vi "Stellglied.vi"(8 "error in (no error)":errorcluster caption="Fehler (Eingang, kein Fehler)", 10 "Stellgröße - Kraft (N)":dbl, 11 "RPDO2 object in":refnum<k20>) -> (0 "error out":errorcluster caption="Fehler (Ausgang)", 3 "Kraft (N)":dbl)   [LabVIEW 2014]
uses:
  <vilib>/CANopenLib/CANOPEN.llb/CANopen Convert To Data [I16].vi
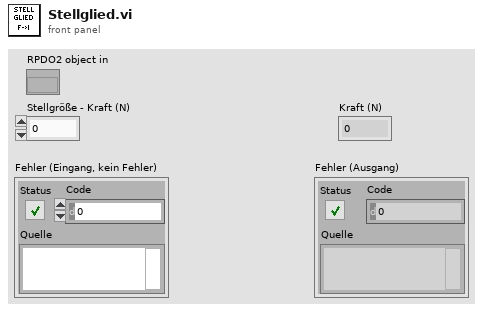
[diagram p1: front panel]
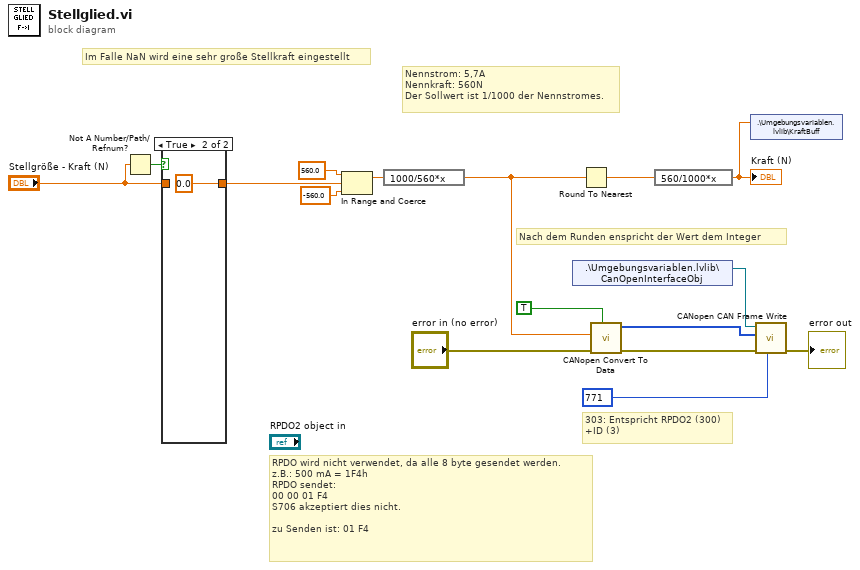
[diagram p0: block diagram]
diagram:
  # "Nennstrom: 5,7A\nNennkraft: 560N\nDer Sollwert ist 1/1000 der Nennstromes."
  # "Im Falle NaN wird eine sehr große Stellkraft eingestellt"
  # "Nach dem Runden enspricht der Wert dem Integer"
  # "RPDO wird nicht verwendet, da alle 8 byte gesendet werden. \nz.B.: 500 mA = 1F4h\nRPDO sendet:\n00 00 01 F4 \nS706 akzeptiert dies nicht.\n\nzu Senden ist: 01 F4"
  # "303: Entspricht RPDO2 (300)\n+ID (3)"
  n1 = Not A Number/Path/Refnum?(number/path/refnum="Stellgröße - Kraft (N)") -> (NaN/Path/Refnum?=w10:bool)
  n2 = case shown="True" w10 {
    tunnel: [w17 0.0 ("Stellgröße - Kraft (N)")] -> w1
    tunnel: "Stellgröße - Kraft (N)" -> [w17 _]
    frame False {
    }
    frame True {
    }
  }
  n3 = In Range and Coerce(upper limit=560.0 ("Obergrenze"), x=w1, lower limit=-560.0 ("Untergrenze")) -> (coerced(x)=w5:dbl)  [unwired: 1 out]
  n4 = expression code="1000/560*x"(w5) -> (w4:dbl)
  n5 = shared-variable ".\\Umgebungsvariablen.lvlib\\CanOpenInterfaceObj"() -> (w13:refnum<k20>)  [unwired: 1 in, 1 out]
  n6 = Round To Nearest(number=w4) -> (nearest integer value=w3:dbl)
  n7 = call-poly <vilib>:"CANopen Convert To Data.vi"("trim"=TRUE, "error in (no error)"="error in (no error)", "signed 16-bit integer"=w4) -> ("error out"=w12:errorcluster, "CANopen data out"=w8:u8[])  [unwired: 7 in]
  n8 = expression code="560/1000*x"(w3) -> (w2:dbl)
  "Kraft (N)" <- w2
  n9 = shared-variable ".\\Umgebungsvariablen.lvlib\\KraftBuff"(w2) -> ()  [unwired: 1 in, 1 out]
  n10 = call <vilib>:"CANopen CAN Frame Write.vi"("COB-ID (0)"=u32 771, "error in (no error)"=w12, "CAN message data"=w8, "interface object  in"=w13) -> ("error out"=→"error out":errorcluster)  [unwired: 6 in, 1 out]
